vi "Configure Channel And Trace.vi"(5 "Active Trace (1)":i32=1, 6 "Data Format (0: Logarithmic Magnitude)":u16(ring) items=["Logarithmic Magnitude", "Phase", "Group Delay", "Smith Chart  Linear (Lin/Phase)", "Smith Chart  Logarithmic (Log/Phase)", "Smith Chart  Complex (Real/Imag)", "Smith Chart  Impedance (R+jX)", "Smith Chart  Admittance (G+jB)", "Polar Format (Linear)", "Polar Format (Logarithmic)", "Polar Format (Re/Im)", "Linear Magnitude", "SWR", "Real", "Imaginary", "Epanded Phase", "Positive Phase"], 7 "Active Channel (1)":i32=1, 8 "error in (no error)":errorcluster, 9 "Measurement Parameters (0: S11)":u16(ring) items=["S11", "S21", "S31", "S41", "S12", "S22", "S32", "S42", "S13", "S23", "S33", "S43", "S14", "S24", "S34", "S44", "A", "B", "C", "D", "R1", "R2", "R3", "R4", "AUX1", "AUX2", "TR", "T", "R"], 10 "Number of Traces (1)":i32=1, 11 "VISA resource name":refnum<visa-resource-name>) -> (0 "error out":errorcluster, 3 "VISA resource name out":refnum<visa-resource-name>)   [LabVIEW 2015, in "Agilent ENA Series.lvlib"]
doc: "This VI sets active channel and trace and configures parameters of active trace."
uses:
  Agilent ENA Series.lvlib
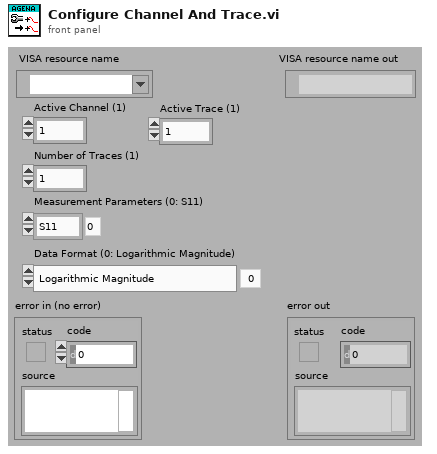
[diagram p1: front panel]
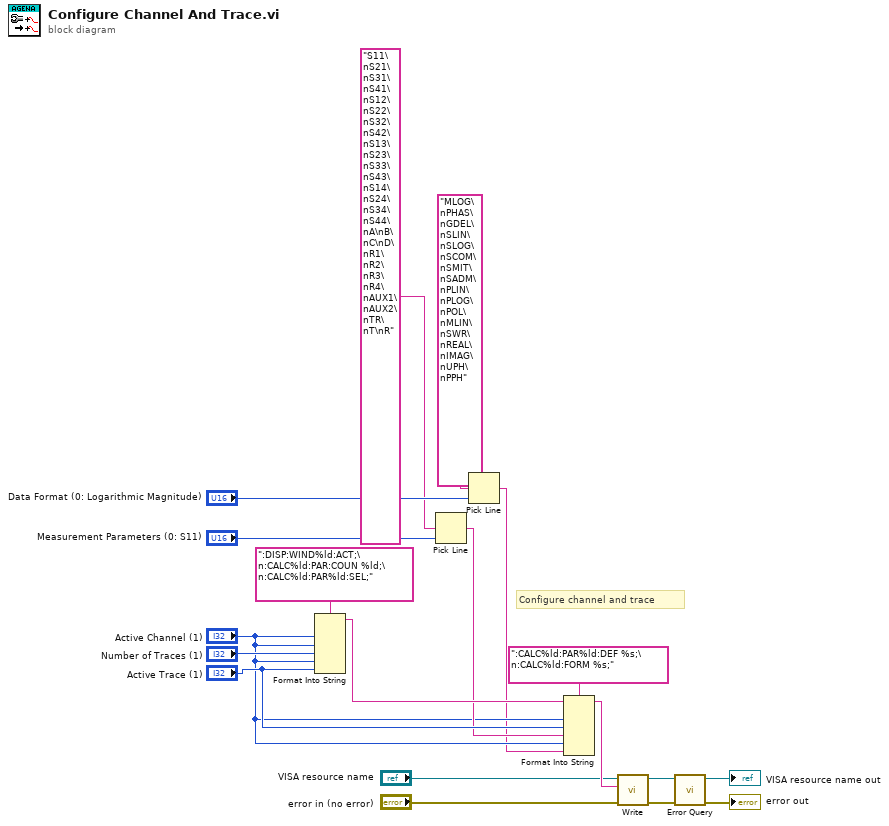
[diagram p0: block diagram]
diagram:
  # "Configure channel and trace"
  n1 = Format Into String(format string=":DISP:WIND%ld:ACT;\n:CALC%ld:PAR:COUN %ld;\n:CALC%ld:PAR%ld:SEL;", "Active Channel (1)", "Active Channel (1)", "Number of Traces (1)", "Active Channel (1)", "Active Trace (1)") -> (resulting string=w5:string)  [unwired: 2 in, 1 out]
  n2 = Pick Line(multi-line string="S11\nS21\nS31\nS41\nS12\nS22\nS32\nS42\nS13\nS23\nS33\nS43\nS14\nS24\nS34\nS44\nA\nB\nC\nD\nR1\nR2\nR3\nR4\nAUX1\nAUX2\nTR\nT\nR", line index="Measurement Parameters (0: S11)") -> (output string=w3:string)  [unwired: 1 in]
  n3 = Pick Line(multi-line string="MLOG\nPHAS\nGDEL\nSLIN\nSLOG\nSCOM\nSMIT\nSADM\nPLIN\nPLOG\nPOL\nMLIN\nSWR\nREAL\nIMAG\nUPH\nPPH" ("string (\"\")"), line index="Data Format (0: Logarithmic Magnitude)") -> (output string=w1:string)  [unwired: 1 in]
  n4 = Format Into String(format string=":CALC%ld:PAR%ld:DEF %s;\n:CALC%ld:FORM %s;", initial string=w5, "Active Channel (1)", "Active Trace (1)", w3, "Active Channel (1)", w1) -> (resulting string=w14:string)  [unwired: 1 in, 1 out]
  n5 = call "Write.vi"("error in (no error)"="error in (no error)", "String ()"=w14, "VISA resource name"="VISA resource name") -> ("error out"=w10:errorcluster, "VISA resource name out"=w11:refnum<visa-resource-name>)  [unwired: 6 in, 1 out]
  n6 = call "Error Query.vi"("error in (no error)"=w10, "VISA resource name"=w11) -> ("error out"=→"error out":errorcluster, "VISA resource name out"=→"VISA resource name out":refnum<visa-resource-name>)  [unwired: 6 in, 2 out]
